vi "AcqData.vi"(5 "Page No":i32, 6 "SPC Memory Config":T1={"Max Block No"=0, "Blocks Per Frame"=1, "Frames Per Page"=1, "Maxpage"=1, "Block Length"=0} {"Frames Per Page" min=1 step=1; "Maxpage" min=1; "Blocks Per Frame" min=1 step=1}, 8 "Error In":errorcluster, 10 "Module No":i16, 11 "DLL Path":path) -> (0 "Error Out":errorcluster, 1 "SingleBlockData":u16[](array[numeric]), 2 "Module No":i16, 3 "DLL Path":path, 4 "MultiBlockData":u16[][](array[numeric]))   [LabVIEW 2019]
doc: "This VI is a wrapper for the SPC_read_data_block.vi calculating the necessary parameters from the 'SPC Memory Config' cluster for convenience.\nThe memory for 'Data Buffer' gets allocated.\nUse the 1D or 2D BlockData output according to your blocks per frame value.\n\n<b>Note:</b> This VI is set to execute as preallocated clone to improve performance when run in parallel loops for multi module setups.\n\ninfo@becker-hickl.com"
uses:
  SPC_Controls/ConfigMem.ctl
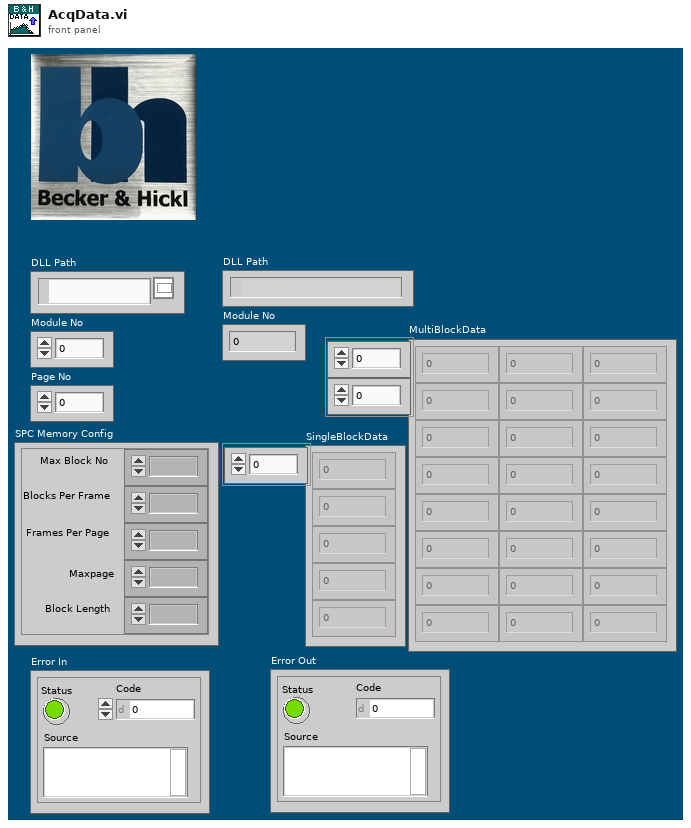
[diagram p1: front panel]
types:
  T1 = typedef "ConfigMem.ctl" = cluster{"Max Block No":i32, "Blocks Per Frame":i32, "Frames Per Page":i32, "Maxpage":i32, "Block Length":i32}
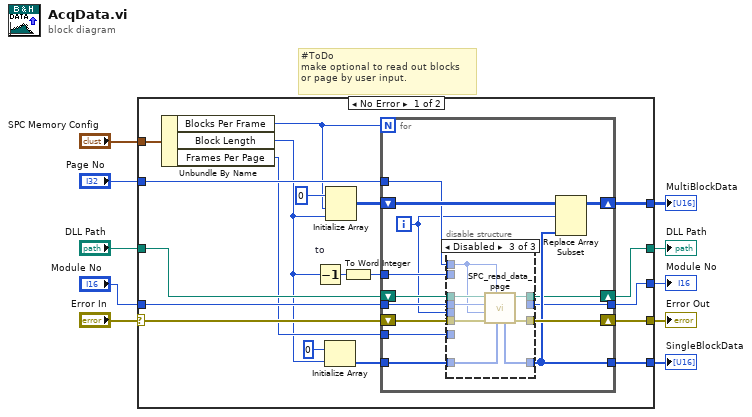
[diagram p0: block diagram]
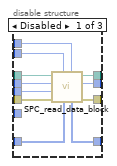
[diagram p2: hidden frame]
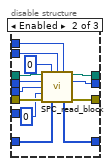
[diagram p3: hidden frame]
diagram:
  # "#ToDo\nmake optional to read out blocks\nor page by user input."
  n1 = case shown="No Error" "Error In" {
    selector: "Error In" -> [w23 w78]
    tunnel: [w29 w78] -> w10
    tunnel: [w28 w77] -> w9
    tunnel: "SPC Memory Config" -> [w21 _]
    tunnel: "Module No" -> [w24 w76]
    tunnel: "DLL Path" -> [w22 w77]
    tunnel: "Page No" -> [w19 _]
    tunnel: [w18 w76] -> w3
    tunnel: [w17 _] -> w2
    tunnel: [w16 _] -> w1
    frame No Error {
      n2 = Unbundle By Name(w21) -> ("Blocks Per Frame"=w12:i32, "Block Length"=w11:i32, "Frames Per Page"=w13:i32)
      n3 = Decrement "to"(x=w11) -> (x-1=w15:i32)
      n4 = Initialize Array(u16 0 ("Element Data"), w11) -> (w20:u16[])
      n5 = Initialize Array(u16 0 ("element"), w12, w11) -> (w25:u16[][])
      n6 = To Word Integer(number=w15) -> (16bit integer=w14:i16)
      n7 = for {
        N: w12 -> [_]
        shift-right: [w35] -> w28
        shift-left: w22 -> [w43]
        shift-right: [w42] -> w29
        shift-left: w23 -> [w41]
        shift-right: [w38] -> w16
        shift-left: w25 -> [w40]
        tunnel: w24 -> [w36]
        tunnel: w19 -> [w34]
        tunnel: [w33] -> w18
        tunnel: w14 -> [w32]
        tunnel: w20 -> [w39]
        tunnel: [w37] -> w17
        tunnel: w13 -> [w31]
        i -> [w30]
        n8 = disable-structure shown="Disabled" {
          disable-tunnel: w43 -> [w54 w65 w74]
          disable-tunnel: [w53 w66 w71] -> w42
          disable-tunnel: w41 -> [w52 w67 w75]
          disable-tunnel: w30 -> [w51 w57 _]
          disable-tunnel: w39 -> [w50 w63 w69]
          disable-tunnel: [w49 w62 w72] -> w37
          disable-tunnel: w36 -> [w48 w58 w73]
          disable-tunnel: [w47 w64 w70] -> w35
          disable-tunnel: w34 -> [w46 w61 w68]
          disable-tunnel: [w45 w56 _] -> w33
          disable-tunnel: w32 -> [w44 w60 _]
          disable-tunnel: w31 -> [_ _ _]
          frame Disabled {
            n9 = call "SPC_read_data_block.vi"("page"=w46, "Data Buffer"=w50, "to"=w44, "Error In"=w52, "block"=w51, "Module No"=w48, "DLL Path"=w54) -> ("Error Out"=w53:errorcluster, "Module No"=w45:i16, "DLL Path"=w47:path, "Data"=w49:u16[])  [unwired: 1 in]
          }
          frame Enabled {
            n10 = call "SPC_read_block.vi"("DLL Path"=w65, "from"=i16 0, "to"=w60, "page"=w61, "Module No"=w58, "block"=w57, "frame"=0, "Error In"=w67, "Data Buffer"=w63) -> ("DLL Path"=w64:path, "Module No"=w56:i16, "Data"=w62:u16[], "Error Out"=w66:errorcluster)  [unwired: 3 in]
          }
          frame Disabled {
            n11 = call "SPC_read_data_page.vi"("DataBuffer"=w69, "First Page"=w68, "Error In"=w75, "Last Page"=w68, "Module No"=w73, "DLL Path"=w74) -> ("Error Out"=w71:errorcluster, "DLL Path"=w70:path, "Output Data"=w72:u16[])  [unwired: 2 in, 1 out]
          }
        }
        n12 = Replace Array Subset(array=w40, new element=w37, index (row)=w30) -> (w38:u16[][])  [unwired: 1 in]
      }
    }
    frame Error {
    }
  }
  "Error Out" <- w10
  "DLL Path" <- w9
  "Module No" <- w3
  "SingleBlockData" <- w2
  "MultiBlockData" <- w1
